vi "PCAN_WRITE.vi"(8 "error in (no error)":errorcluster, 11 "TPCANMsg":T1={"ID"=0, "MSGTYPE"=128, "LEN"=0, "Data"=[]} {"MSGTYPE" items=["STATUS"=128, "EXTENDED"=2, "RTR"=1, "DATA MSG"=0]}) -> (0 "error out":errorcluster, 3 "error":T2 items=["CAN_ERR_OK"=0, "CAN_ERR_XMTFULL"=1, "CAN_ERR_OVERRUN"=2, "CAN_ERR_BUSLIGHT"=4, "CAN_ERR_BUSHEAVY"=8, "CAN_ERR_BUSOFF"=16, "CAN_ERR_QRCVEMPTY"=32, "CAN_ERR_QOVERRUN"=64, "CAN_ERR_QXMTFULL"=128, "CAN_ERR_REGTEST"=256, "CAN_ERR_NOVXD"=512, "CAN_ERR_RESOURCE"=8192, "CAN_ERR_ILLPARAMTYPE"=16384, "CAN_ERR_ILLPARAMVAL"=32768])   [LabVIEW 2016]
doc: "///////////////////////////////////////////////////////////////////////////////\n// CAN_Write()\n// Schreibt eine Message \n// moegliche Fehler: NOVXD RESOURCE BUSOFF QXMTFULL\n//\n\nDWORD __stdcall CAN_Write( TPCANMsg* pMsgBuff);"
uses:
  PCAN_ERROR.ctl
  PCAN_USB.DLL
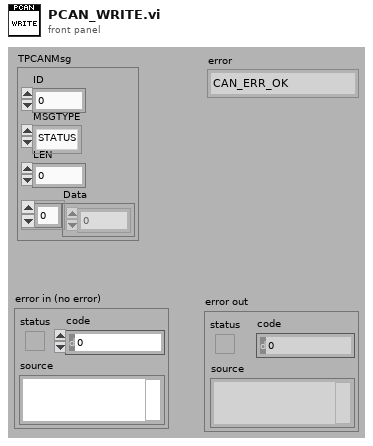
[diagram p1: front panel]
types:
  T1 = cluster{"ID":u32, "MSGTYPE":u8, "LEN":u8, "Data":u8[]}
  T2 = typedef "PCAN_ERROR.ctl" = i32
  T3 = enum16{"big-endian, network order", "native, host order", "little-endian"}
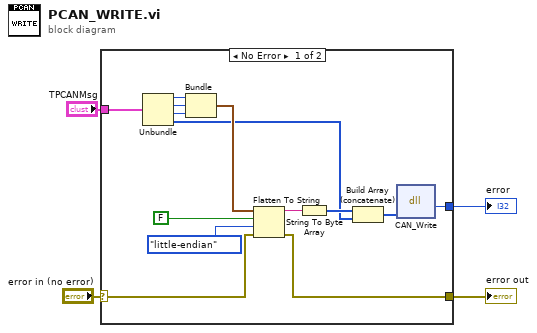
[diagram p0: block diagram]
diagram:
  n1 = case shown="No Error" "error in (no error)" {
    selector: "error in (no error)" -> [w6 w19]
    tunnel: [w18 _] -> w2
    tunnel: [w5 w19] -> w3
    tunnel: "TPCANMsg" -> [w17 _]
    frame No Error {
      n2 = Unbundle(w17) -> ("ID"=w16:u32, "MSGTYPE"=w15:u8, "LEN"=w14:u8, "Data"=w10:u8[])
      n3 = Bundle("ID"=w16, "MSGTYPE"=w15, "LEN"=w14) -> (w13:cluster{"ID":u32, "MSGTYPE":u8, "LEN":u8})  [unwired: 1 out]
      n4 = Flatten To String(anything=w13, prepend array or string size? (T)=FALSE, byte order (0:big-endian, network order)=T3."little-endian", error in (no error)=w6) -> (data string=w12:string, error out=w5:errorcluster)  [unwired: 1 out]
      n5 = String To Byte Array(string=w12) -> (unsigned byte array=w11:u8[])
      n6 = Build Array (concatenate)(w11, w10) -> (w9:u8[])
      n7 = dll-call lib="D:/LabView/08_PCAN&Measurement/PCAN_Driver/PCAN_USB.DLL" fn="CAN_Write"("pMsgBuff"=w9) -> ("return type"=w18:i32)  [unwired: 4 in, 2 out]
    }
    frame Error {
    }
  }
  "error out" <- w3
  "error" <- w2
